vi "SIne Wave Generator.vi"(9 "Sampling rate":dbl format="%#_13g", 10 "Frequency":dbl format="%#_13g", 11 "Duration":dbl format="%#_13g") -> (2 "output cluster":cluster{dbl, dbl, dbl[]}, 3 "Array":dbl[](array[numeric]))   [LabVIEW 2021]
uses:
  <vilib>/Analysis/1siggen.llb/Ramp Pattern by Samples.vi
  <vilib>/Analysis/NI_AALBase.lvlib
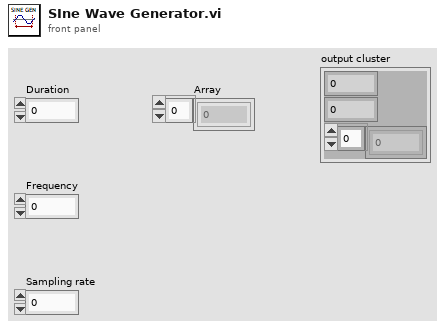
[diagram p1: front panel]
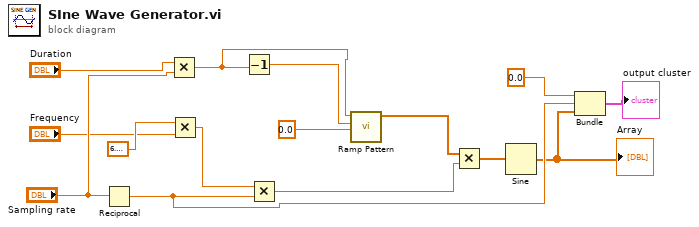
[diagram p0: block diagram]
diagram:
  n1 = Reciprocal(x="Sampling rate") -> (1/x=w3:dbl)
  n2 = Multiply(x="Duration", y="Sampling rate") -> (x*y=w11:dbl)
  n3 = Multiply(x=6.283185307179586, y="Frequency") -> (x*y=w8:dbl)
  n4 = Decrement(x=w11) -> (x-1=w10:dbl)
  n5 = Multiply(x=w8, y=w3) -> (x*y=w14:dbl)
  n6 = call-poly <vilib>:"Ramp Pattern.vi"("start"=0.0, "end"=w10, "samples"=w11) -> ("Ramp Pattern"=w13:dbl[])  [unwired: 7 in, 1 out]
  n7 = Multiply(x=w13, y=w14) -> (x*y=w15:dbl[])
  n8 = Sine(x=w15) -> (sin(x)=w2:dbl[])
  "Array" <- w2
  n9 = Bundle(0.0, w3, w2) -> (→"output cluster":cluster{dbl, dbl, dbl[]})  [unwired: 1 in]
